vi "AudioTest.SoundCheck Data Log Graph Window - Composite.vi"() -> ()   [LabVIEW 2018]
uses:
  TypeDefs/AudioTest.Analysis Data Record.ctl
  TypeDefs/AudioTest.Analysis Folder Navigation Status.ctl
  <vilib>/KATE/Queues/Queue Utils.lvlib
  <vilib>/KATE/Files/File Utils.lvlib
panel:
  in  "Main Tab":enum32{"Data", "Setup"}(tab)
  out "Comment":string
  out "Count":i32
  out "Index":i32
  out "TopEnd":bool
  out "BotEnd":bool
  out "Loc":string
  out "Result":string
  out "Description":string
  out "Result Code":i32 caption="Code"
  out "Folder":string
  in  "UUTDir Next":bool
  in  "UUTDir Prev":bool
  in  "Snapshot":bool
  out "Name 1 1":string
  out "Graph1 1":cluster{"X":dbl[], "Y":dbl[]}[](graph)
  out "Graph1 2":cluster{"X":dbl[], "Y":dbl[]}[](graph)
  out "Name 1 2":string
  out "Name 3 3":string
  out "Graph3 3":cluster{"X":dbl[], "Y":dbl[]}[](graph)
  out "Name 3 2":string
  out "Graph3 2":cluster{"X":dbl[], "Y":dbl[]}[](graph)
  out "Name 3 1":string
  out "Graph3 1":cluster{"X":dbl[], "Y":dbl[]}[](graph)
  out "Name 2 4":string
  out "Graph2 4":cluster{"X":dbl[], "Y":dbl[]}[](graph)
  out "Graph2 3":cluster{"X":dbl[], "Y":dbl[]}[](graph)
  out "Name 2 3":string
  out "Graph2 2":cluster{"X":dbl[], "Y":dbl[]}[](graph)
  out "Name 2 2":string
  out "Graph2 1":cluster{"X":dbl[], "Y":dbl[]}[](graph)
  out "Name 2 1":string
  out "Graph1 4":cluster{"X":dbl[], "Y":dbl[]}[](graph)
  out "Name 1 4":string
  out "Graph1 3":cluster{"X":dbl[], "Y":dbl[]}[](graph)
  out "Name 1 3":string
  out "Left Level":string caption="Level"
  out "Right Level":string caption="Level"
  out "Mic Level":string caption="Level"
  out "Mic Covered Level":string caption="Covered"
  in  "Graphs":T1[](array[typedef])
  in  "QName":string="Plot_Composite"
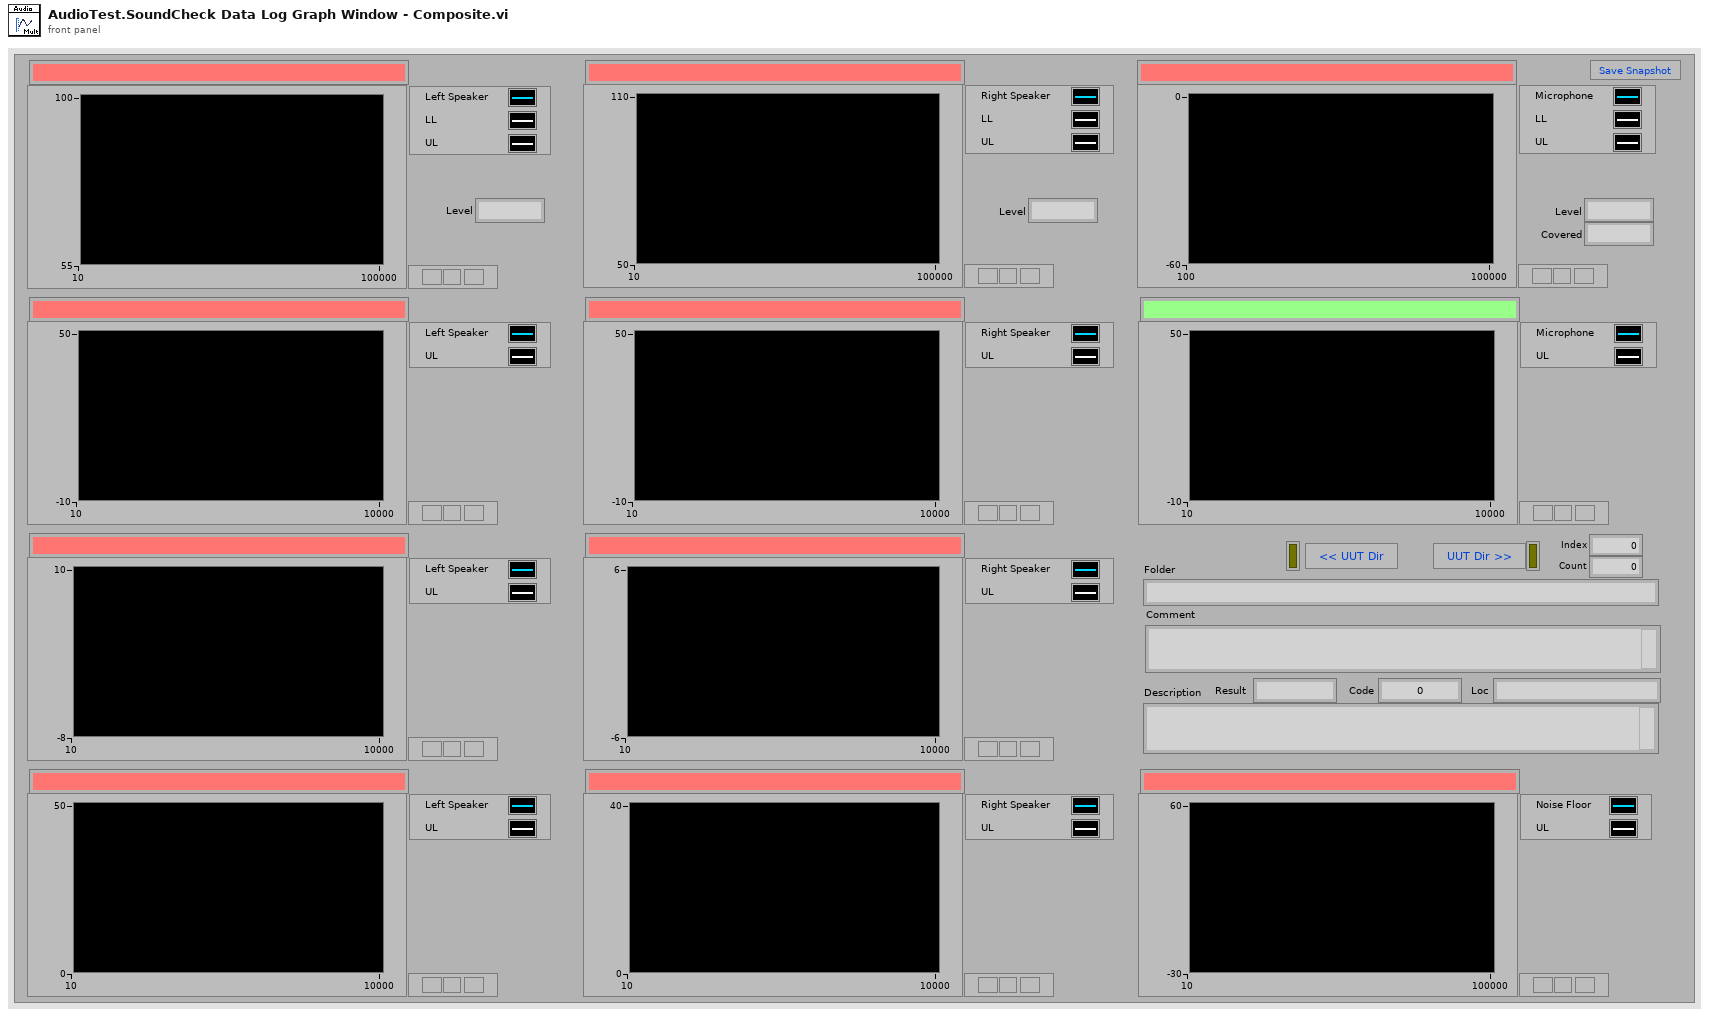
[diagram p1: front panel]
types:
  T1 = typedef "AudioTest.Analysis Data Record.ctl" = cluster{"Name":string, "X Units":string, "Y Units":string, "DataPlots":cluster{"X":dbl[], "Y":dbl[]}[], "LimitPlots":cluster{"X":dbl[], "Y":dbl[]}[], "DataPlotNames":string[], "LimitPlotNames":string[], "Fail":bool}
  T2 = typedef "imagedata.ctl" = cluster{"image type":i32, "image depth":i32, "image":u8[], "mask":u8[], "colors":u32[], "Rectangle":cluster{"left":i16, "top":i16, "right":i16, "bottom":i16}}
  T3 = enum32{"Invalid", "Standard", "Closed", "Hidden", "Minimized", "Maximized"}
  T4 = typedef "AudioTest.Analysis Folder Navigation Status.ctl" = cluster{"Index":i32, "Count":i32, "HightEnd":bool, "LowtEnd":bool}
  T5 = cluster{"Graphs":T1[], "PlotColors":u32[], "LimColors":u32[]}
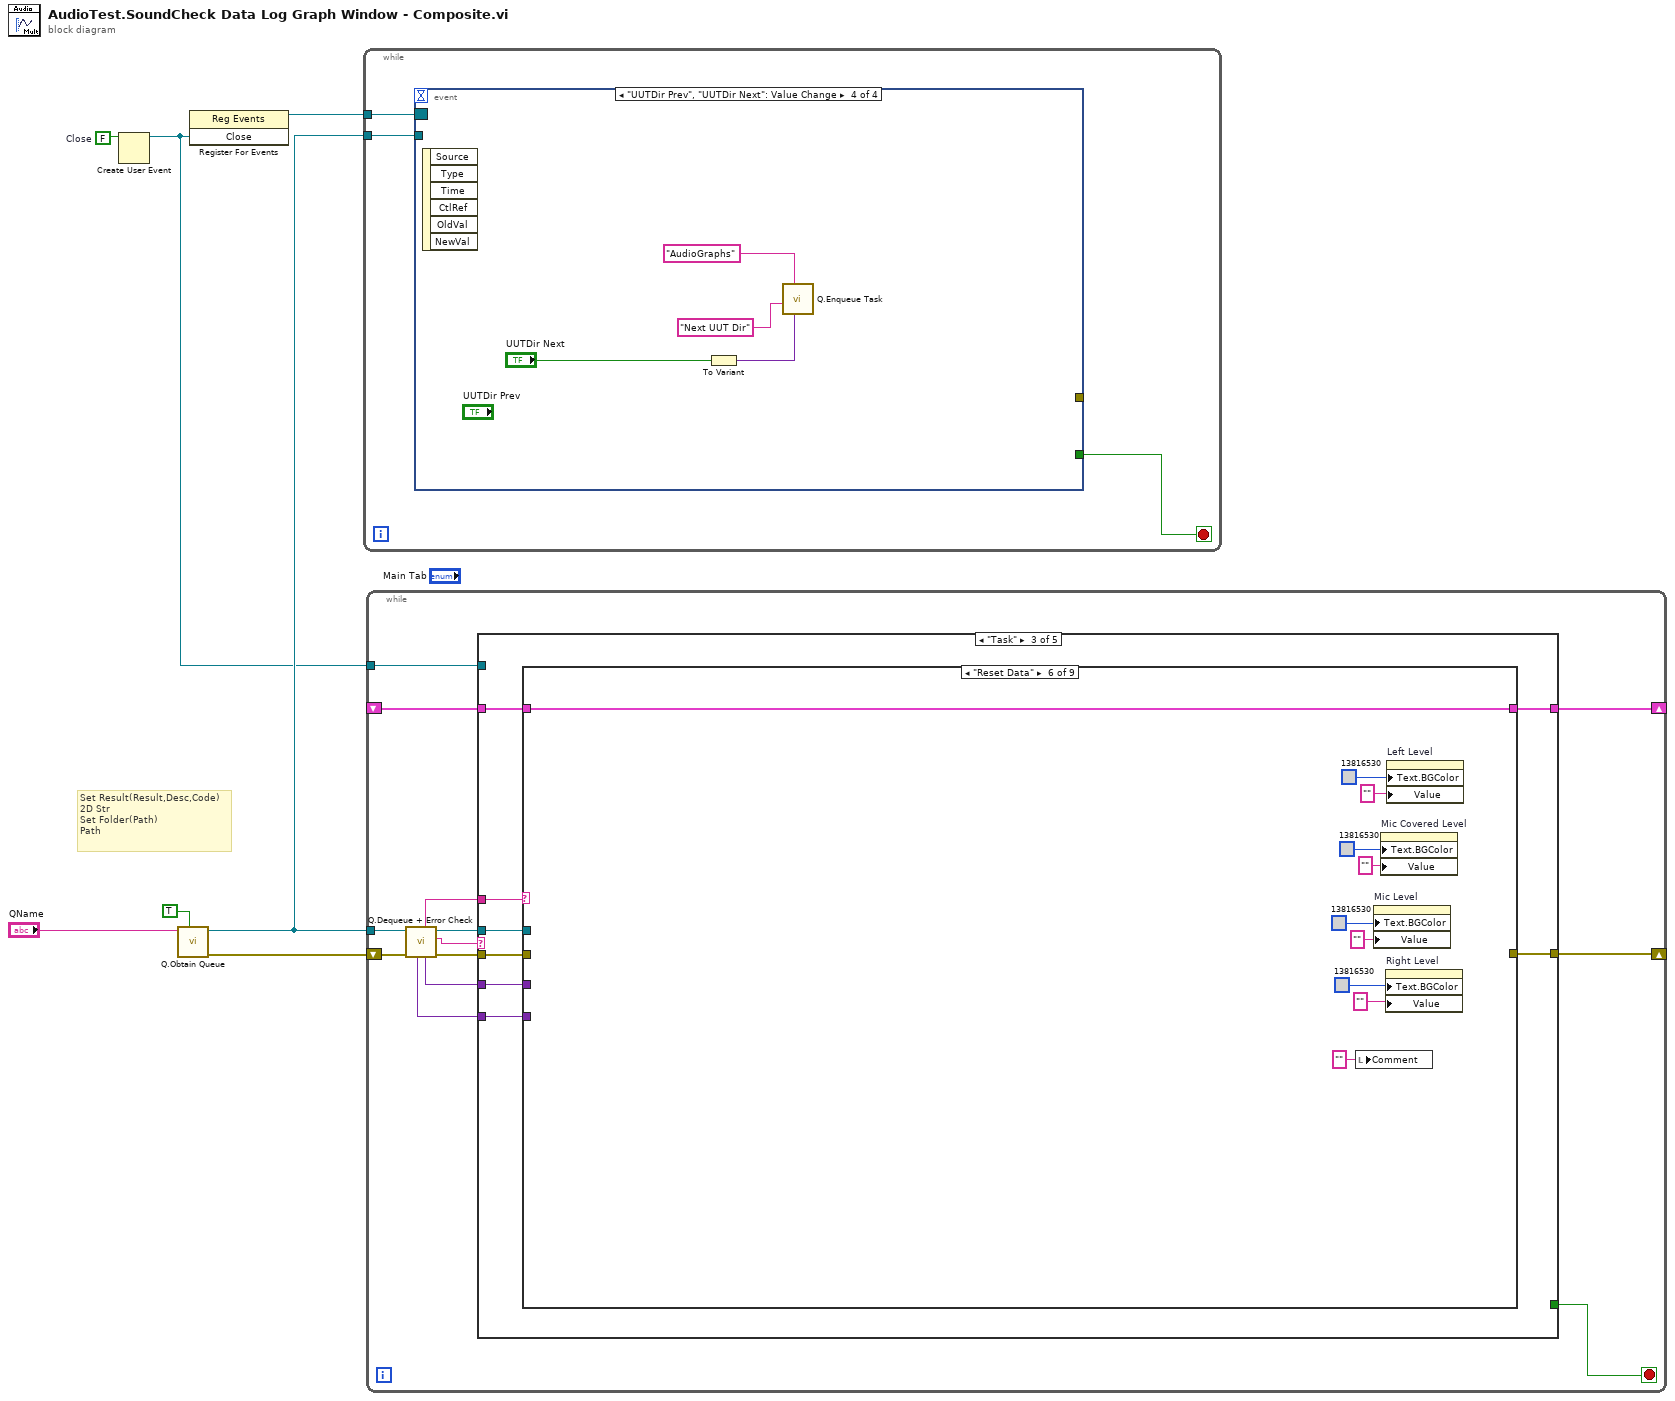
[diagram p0: block diagram]
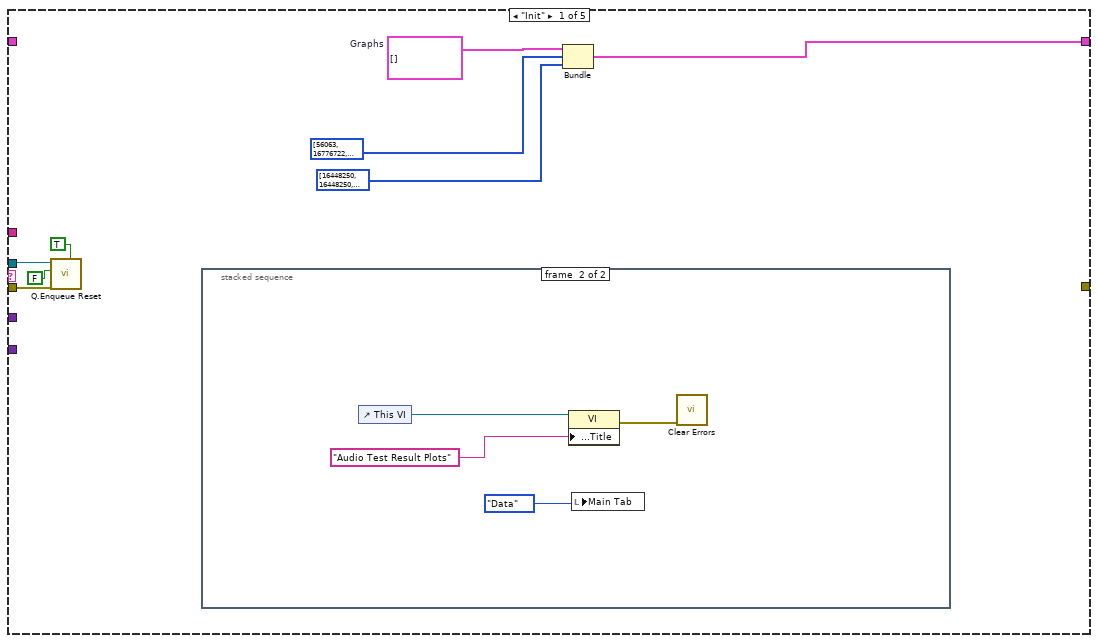
[diagram p2: hidden frame]
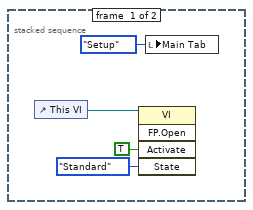
[diagram p3: hidden frame]
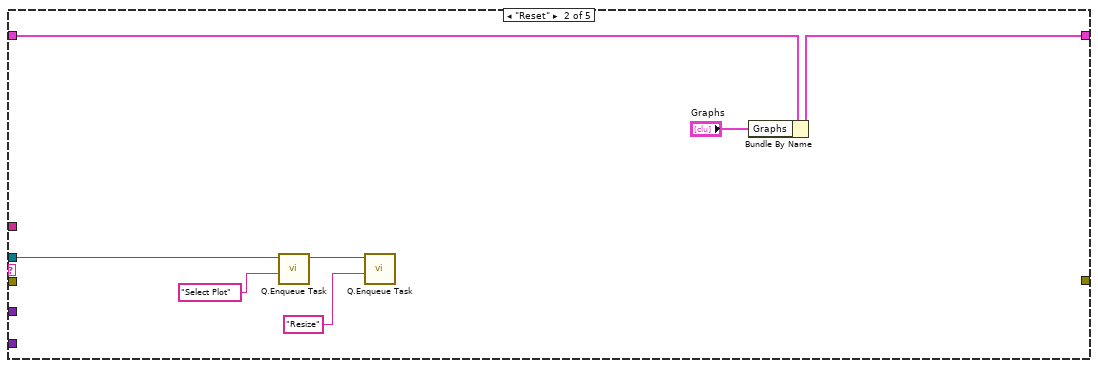
[diagram p4: hidden frame]
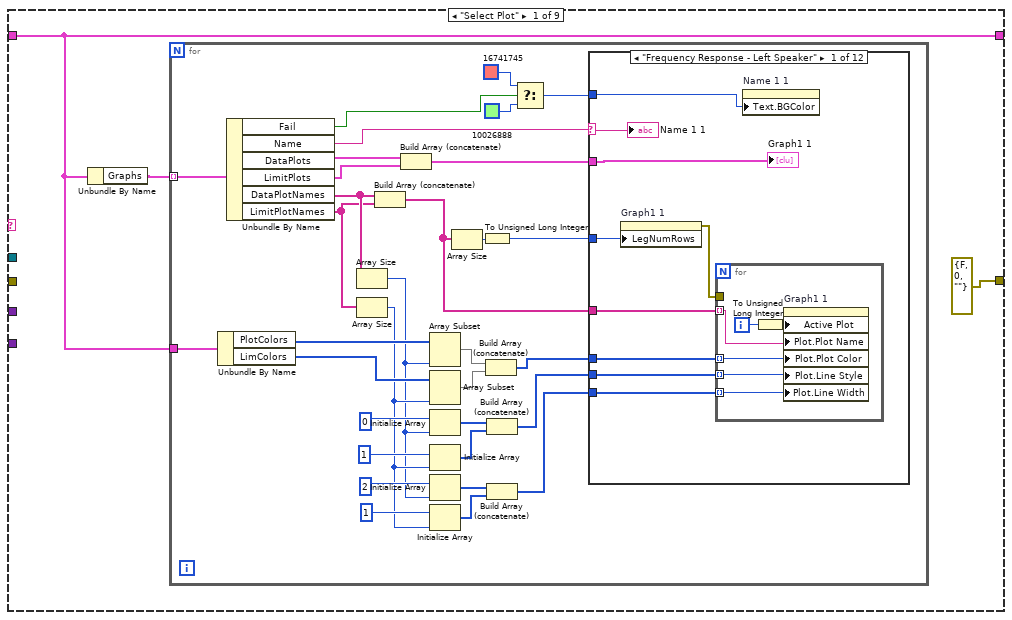
[diagram p5: hidden frame]
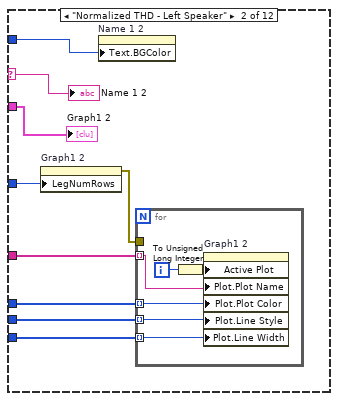
[diagram p6: hidden frame]
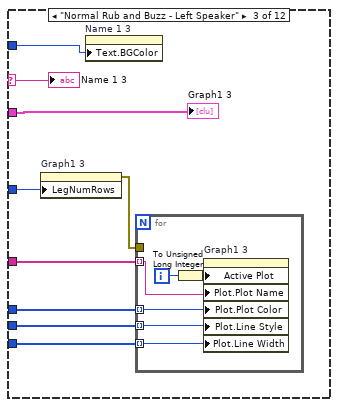
[diagram p7: hidden frame]
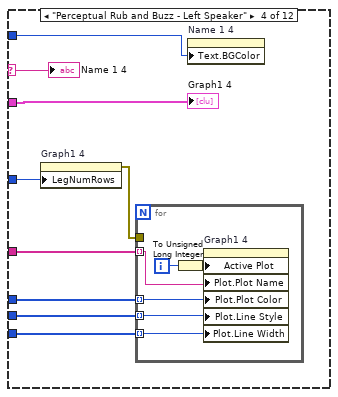
[diagram p8: hidden frame]
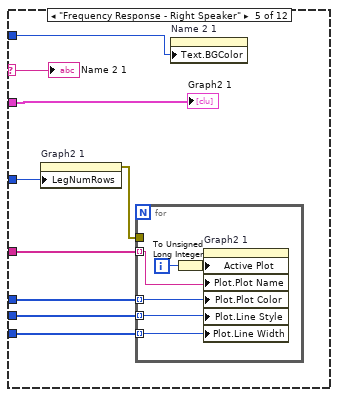
[diagram p9: hidden frame]
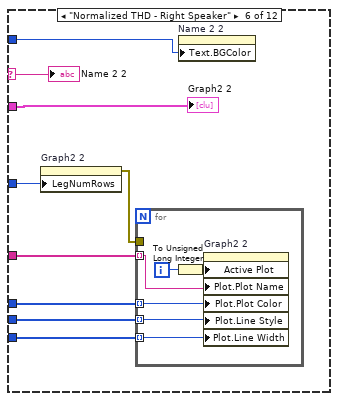
[diagram p10: hidden frame]
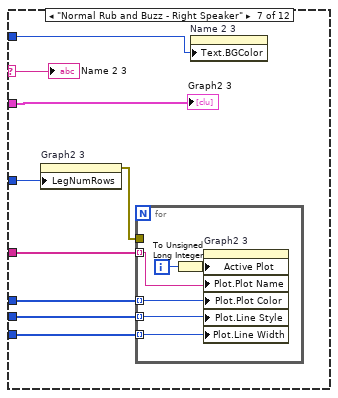
[diagram p11: hidden frame]
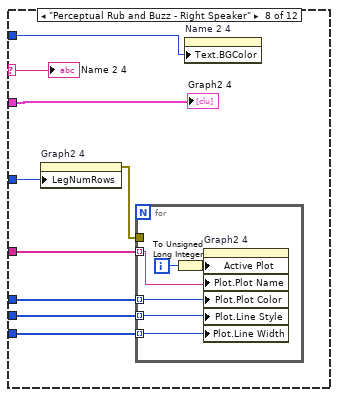
[diagram p12: hidden frame]
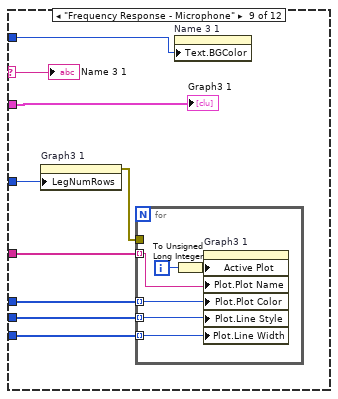
[diagram p13: hidden frame]
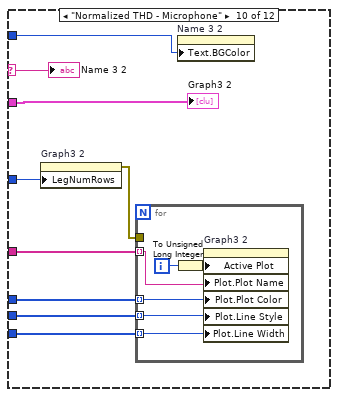
[diagram p14: hidden frame]
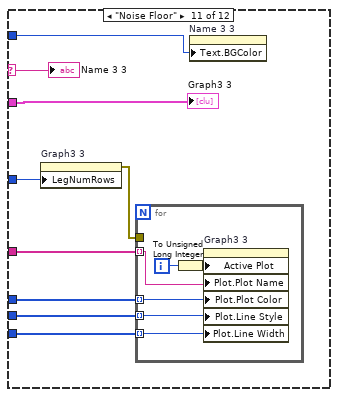
[diagram p15: hidden frame]
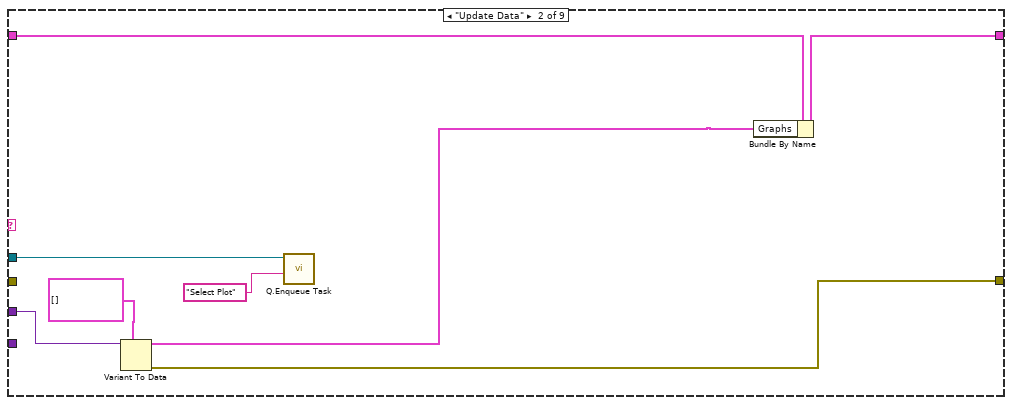
[diagram p17: hidden frame]
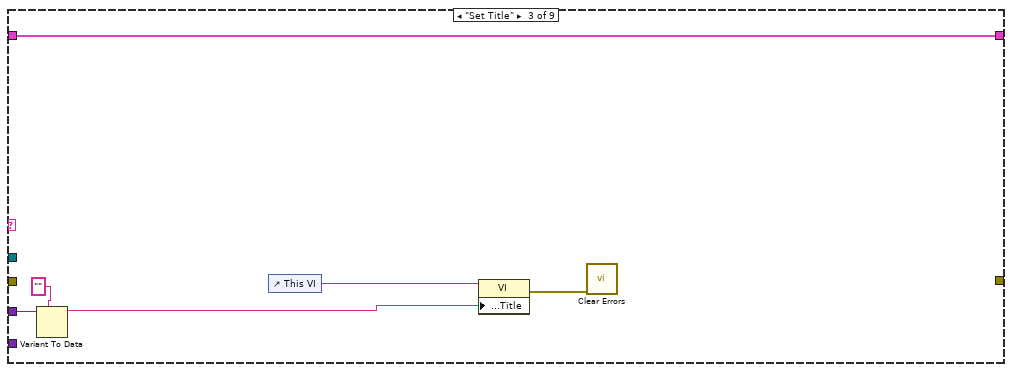
[diagram p18: hidden frame]
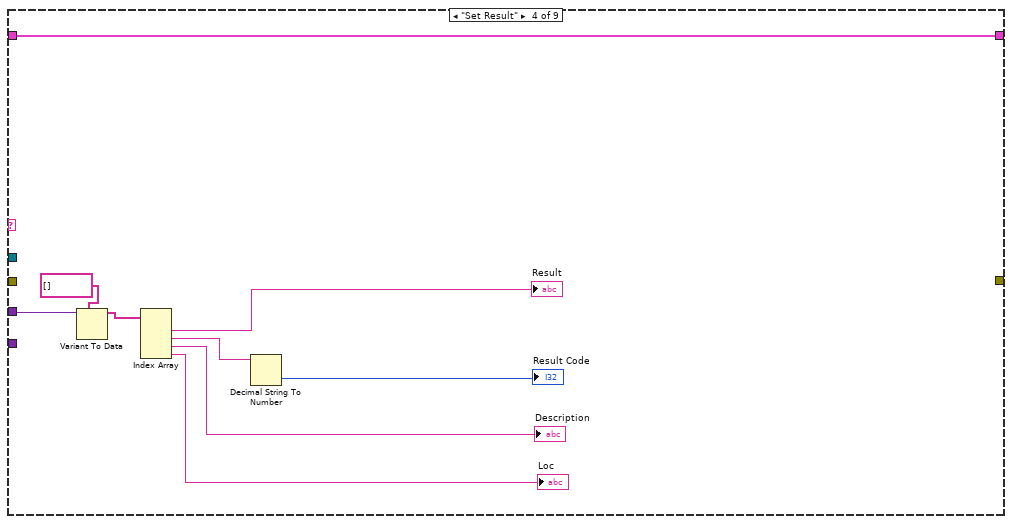
[diagram p19: hidden frame]
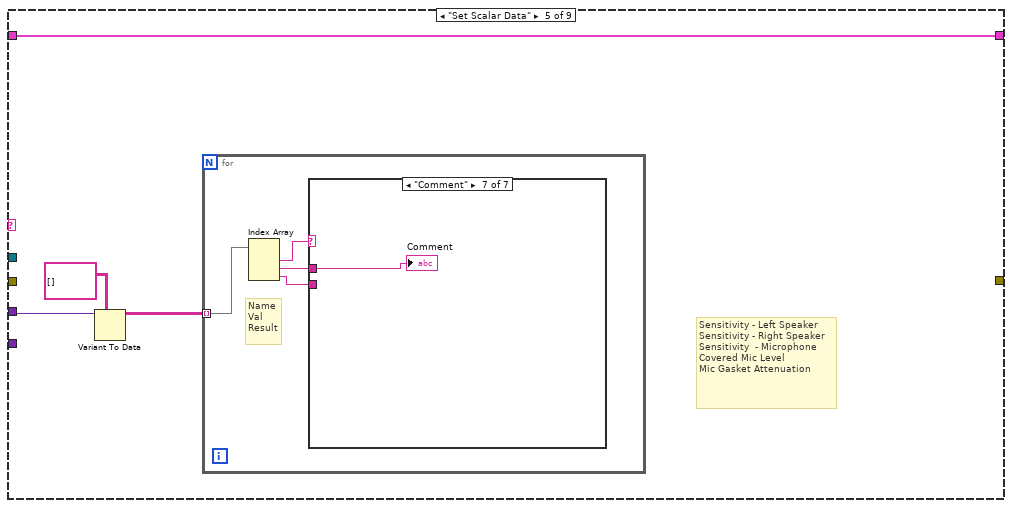
[diagram p20: hidden frame]
diagram:
  w7 = FALSE  # Close
  # "Set Result(Result,Desc,Code)\n2D Str\nSet Folder(Path)\nPath"
  n1 = Create User Event(user event datatype=w7) -> (user event=w2:refnum<user-event>)  [unwired: 1 in, 1 out]
  n2 = call <vilib>:"Q.Obtain Queue.vi"("Enqueue Init"=TRUE, "Q Name"="QName") -> ("error out"=w4:errorcluster, "Q Out"=w3:refnum<queue>)  [unwired: 7 in, 1 out]
  n3 = register-events(w2) -> (reference out=w6:refnum<event-registration>)  [unwired: 2 in, 1 out]
  n4 = while {
    tunnel: w6 -> [w10]
    tunnel: w3 -> [w9]
    stop <- w8 stop-if-true
    n5 = event shown="[3] \"UUTDir Prev\", \"UUTDir Next\": Value Change" {
      selector: w10 -> [_ _ _ _]
      dyn-events: _ -> [_ _ _ _]
      timeout: _ -> [_ _ _ _]
      tunnel: w9 -> [w13 w16 _ _]
      tunnel: [TRUE TRUE _ _] -> w8
      tunnel: [_ _ w23 _] -> _
      event Panel Close? {
        n6 = event-data() -> ()  [unwired: 1 in, 4 out]
        n7 = call <vilib>:"Q.Enqueue Exit.vi"("Q In"=w13) -> ("error out"=w12:errorcluster)  [unwired: 9 in, 1 out]
        n8 = call <vilib>:"Clear Errors.vi"("error in (no error)"=w12) -> ()  [unwired: 5 in, 2 out]
        n9 = event-data("Discard?"=TRUE) -> ()  [unwired: 1 in, 1 out]
      }
      event User Event {
        n10 = event-data() -> ()  [unwired: 1 in, 4 out]
        n11 = call <vilib>:"Q.Enqueue Exit.vi"("Q In"=w16) -> ("error out"=w15:errorcluster)  [unwired: 9 in, 1 out]
        n12 = call <vilib>:"Clear Errors.vi"("error in (no error)"=w15) -> ()  [unwired: 5 in, 2 out]
      }
      event "Snapshot": Value Change {
        n13 = event-data() -> ()  [unwired: 1 in, 6 out]
        n14 = control-ref of="This VI"() -> (w27:refnum<vi>)
        n15 = invoke class="VI" method="FP.Get Image"(reference=w27, "visible area only"=FALSE ("Visible Area Only"), "image depth"=24 ("Image Depth")) -> ("image data"=w24:T2)  [unwired: 3 in, 5 out]
        n16 = call "File Dialog"("prompt"="Select path to save screen shot", "default name"="Audio Graphs.png", "pattern (all files)"="*.png") -> ("selected path"=w22:path, "cancelled"=w18:bool)  [unwired: 9 in, 2 out]
        n17 = case shown="False" w18 {
          tunnel: w24 -> [w30 _]
          tunnel: [w29 _] -> w23
          tunnel: w22 -> [w28 _]
          frame False {
            n18 = call <vilib>:"Write PNG File.vi"("image data"=w30, "path to PNG file"=w28) -> ("error out"=w29:errorcluster)  [unwired: 8 in, 1 out]
          }
          frame True {
          }
        }
      }
      event "UUTDir Prev", "UUTDir Next": Value Change {
        n19 = event-data() -> ()  [unwired: 1 in, 6 out]
        n20 = To Variant(anything="UUTDir Next") -> (Variant=w32:variant)
        n21 = call <vilib>:"Q.Enqueue Task.vi"("Data1"=w32, "Q Name"="AudioGraphs", "Task Name"="Next UUT Dir") -> ()  [unwired: 7 in, 2 out]
      }
    }
  }
  n22 = while {
    shift-right: [w39] -> _
    shift-left: w4 -> [w44]
    tunnel: w3 -> [w42]
    shift-right: [w37] -> _
    shift-left: _ -> [w36]
    tunnel: w2 -> [w35]
    stop <- w38 stop-if-true
    n23 = call <vilib>:"Q.Dequeue + Error Check.vi"("Error In"=w44, "Q In"=w42) -> ("error out"=w45:errorcluster, "Cmd"=w47:string, "Q Out"=w46:refnum<queue>, "Data1"=w41:variant, "Sub"=w43:string, "Data2"=w40:variant)  [unwired: 4 in]
    n24 = case shown="\"Task\"" w47 {
      tunnel: w46 -> [w55 w68 w77 _ w372]
      tunnel: w45 -> [w54 _ w76 _ _]
      tunnel: w43 -> [_ _ w78 _ _]
      tunnel: w41 -> [_ _ w75 _ _]
      tunnel: w40 -> [_ _ w74 _ _]
      tunnel: [_ _ w71 _ _] -> w39
      tunnel: [_ _ _ _ TRUE] -> w38
      tunnel: [w49 w70 w72 w369 w376] -> w37
      tunnel: w36 -> [_ w69 w73 w370 w376]
      tunnel: w35 -> [_ _ _ _ w375]
      frame "Init" {
        w52 = T1[] []  # Graphs
        n25 = call <vilib>:"Q.Enqueue Reset.vi"("Top of Q(T)"=TRUE, "Error In"=w54, "Flush Queue(T)"=FALSE, "Q In"=w55) -> ()  [unwired: 6 in, 2 out]
        n26 = stacked-sequence {
          frame #0 {
            n27 = control-ref of="This VI"() -> (w59:refnum<vi>)
            n28 = invoke class="VI" method="FP.Open"(reference=w59, "Activate"=TRUE ("Activate?"), "State"=T3."Standard") -> ()  [unwired: 2 in, 5 out]
            n29 = local write "Main Tab"(enum32{"Data", "Setup"}."Setup" ("Main Tab")) -> ()
          }
          frame #1 {
            n30 = control-ref of="This VI"() -> (w63:refnum<vi>)
            n31 = property class="VI"(reference=w63, "Front Panel.Title"="Audio Test Result Plots") -> (error out=w62:errorcluster)  [unwired: 1 in, 1 out]
            n32 = local write "Main Tab"(enum32{"Data", "Setup"}."Data" ("Main Tab")) -> ()
            n33 = call <vilib>:"Clear Errors.vi"("error in (no error)"=w62) -> ()  [unwired: 5 in, 2 out]
          }
        }
        n34 = Bundle("Graphs"=w52, "PlotColors"=u32[] [56063, 16776722, 16730898, 16711925, 6618880], "LimColors"=u32[] [16448250, 16448250, 16448250, 16448250, 16448250, 16448250]) -> (w49:T5)  [unwired: 1 in]
      }
      frame "Reset" {
        n35 = call <vilib>:"Q.Enqueue Task.vi"("Task Name"="Select Plot", "Q In"=w68) -> ("Q Out"=w65:refnum<queue>)  [unwired: 8 in, 1 out]
        n36 = call <vilib>:"Q.Enqueue Task.vi"("Task Name"="Resize", "Q In"=w65) -> ()  [unwired: 8 in, 2 out]
        n37 = Bundle By Name(cluster=w69, "Graphs"="Graphs") -> (w70:T5)
      }
      frame "Task" {
        n38 = case shown="\"Reset Data\"" w78 {
          tunnel: w77 -> [_ w285 _ _ _ _ _ _ _]
          tunnel: w76 -> [_ _ _ _ _ _ _ _ _]
          tunnel: w75 -> [_ w282 w289 w300 w302 _ w346 w363 _]
          tunnel: w74 -> [_ _ _ _ _ _ _ _ _]
          tunnel: w73 -> [w81 w284 w292 w301 w305 w340 w347 w365 w366]
          tunnel: [w81 w283 w292 w301 w305 w340 w347 w365 w366] -> w72
          tunnel: [errorcluster {"status"=FALSE, "code"=0, "source"=""} ("error constant") w281 _ _ _ _ _ _ _] -> w71
          frame "Select Plot" {
            n39 = Unbundle By Name(w81) -> ("Graphs"=w79:T1[])
            n40 = for {
              tunnel: w81 -> [w108]
              tunnel: w79 -> [w87] mode=indexing
              n41 = Unbundle By Name(w108) -> ("PlotColors"=w105:u32[], "LimColors"=w104:u32[])
              n42 = Unbundle By Name(w87) -> ("Fail"=w83:bool, "Name"=w86:string, "DataPlots"=w113:cluster{"X":dbl[], "Y":dbl[]}[], "LimitPlots"=w112:cluster{"X":dbl[], "Y":dbl[]}[], "DataPlotNames"=w107:string[], "LimitPlotNames"=w106:string[])
              n43 = Array Size(array=w107) -> (size(s)=w90:i32)
              n44 = Array Size(array=w106) -> (size(s)=w91:i32)
              n45 = Build Array (concatenate)(w107, w106) -> (w109:string[])
              n46 = Build Array (concatenate)(w113, w112) -> (w88:cluster{"X":dbl[], "Y":dbl[]}[])
              n47 = Array Subset(array=w105, length=w90) -> (w103:u32[])  [unwired: 1 in]
              n48 = Array Subset(array=w104, length=w91) -> (w102:u32[])  [unwired: 1 in]
              n49 = Initialize Array(u8 0 ("Plot.Line Style"), w90) -> (w98:u8[])
              n50 = Initialize Array(u8 1 ("Plot.Line Style"), w91) -> (w97:u8[])
              n51 = Initialize Array(u8 2 ("Plot.Line Style"), w90) -> (w94:u8[])
              n52 = Initialize Array(u8 1 ("Plot.Line Style"), w91) -> (w95:u8[])
              n53 = Array Size(array=w109) -> (size(s)=w111:i32)
              n54 = To Unsigned Long Integer(number=w111) -> (unsigned 32bit integer=w110:u32)
              n55 = Build Array (concatenate)(w103, w102) -> (w101:u32[])
              n56 = Build Array (concatenate)(w98, w97) -> (w96:u8[])
              n57 = Build Array (concatenate)(w94, w95) -> (w89:u8[])
              n58 = Select(t=u32 16741745, s=w83, f=u32 10026888) -> (s? t:f=w82:u32)
              n59 = case shown="\"Frequency Response - Left Speaker\"" w86 {
                selector: w86 -> [w115 w130 w145 w160 w175 w190 w205 w220 w235 w250 w265 _]
                tunnel: w110 -> [w122 w137 w152 w167 w182 w197 w212 w227 w242 w257 w272 _]
                tunnel: w109 -> [w120 w135 w150 w165 w180 w195 w210 w225 w240 w255 w270 _]
                tunnel: w101 -> [w119 w134 w149 w164 w179 w194 w209 w224 w239 w254 w269 _]
                tunnel: w96 -> [w118 w133 w148 w163 w178 w193 w208 w223 w238 w253 w268 _]
                tunnel: w89 -> [w117 w132 w147 w162 w177 w192 w207 w222 w237 w252 w267 _]
                tunnel: w88 -> [w116 w131 w146 w161 w176 w191 w206 w221 w236 w251 w266 _]
                tunnel: w82 -> [w114 w129 w144 w159 w174 w189 w204 w219 w234 w249 w264 _]
                frame "Frequency Response - Left Speaker" {
                  n60 = property on="Graph1 1" class="XYGraph (strict)"("LegNumRows"=w122) -> (error out=w121:errorcluster)  [unwired: 2 in, 1 out]
                  n61 = for {
                    tunnel: w120 -> [w126] mode=indexing
                    tunnel: w121 -> [_]
                    tunnel: w119 -> [w125] mode=indexing
                    tunnel: w118 -> [w124] mode=indexing
                    tunnel: w117 -> [w123] mode=indexing
                    i -> [w127]
                    n62 = To Unsigned Long Integer(number=w127) -> (unsigned 32bit integer=w128:u32)
                    n63 = property on="Graph1 1" class="XYGraph (strict)"("Active Plot"=w128, "Plot.Plot Name"=w126, "Plot.Plot Color"=w125, "Plot.Line Style"=w124, "Plot.Line Width"=w123) -> ()  [unwired: 2 in, 2 out]
                  }
                  n64 = property on="Name 1 1" class="Str"("Text.BGColor"=w114) -> ()  [unwired: 2 in, 2 out]
                  "Graph1 1" <- w116
                  "Name 1 1" <- w115
                }
                frame "Normalized THD - Left Speaker" {
                  n65 = property on="Graph1 2" class="XYGraph (strict)"("LegNumRows"=w137) -> (error out=w136:errorcluster)  [unwired: 2 in, 1 out]
                  n66 = property on="Name 1 2" class="Str"("Text.BGColor"=w129) -> ()  [unwired: 2 in, 2 out]
                  n67 = for {
                    tunnel: w135 -> [w141] mode=indexing
                    tunnel: w136 -> [_]
                    tunnel: w134 -> [w140] mode=indexing
                    tunnel: w133 -> [w139] mode=indexing
                    tunnel: w132 -> [w138] mode=indexing
                    i -> [w142]
                    n68 = To Unsigned Long Integer(number=w142) -> (unsigned 32bit integer=w143:u32)
                    n69 = property on="Graph1 2" class="XYGraph (strict)"("Active Plot"=w143, "Plot.Plot Name"=w141, "Plot.Plot Color"=w140, "Plot.Line Style"=w139, "Plot.Line Width"=w138) -> ()  [unwired: 2 in, 2 out]
                  }
                  "Graph1 2" <- w131
                  "Name 1 2" <- w130
                }
                frame "Normal Rub and Buzz - Left Speaker" {
                  n70 = property on="Graph1 3" class="XYGraph (strict)"("LegNumRows"=w152) -> (error out=w151:errorcluster)  [unwired: 2 in, 1 out]
                  n71 = property on="Name 1 3" class="Str"("Text.BGColor"=w144) -> ()  [unwired: 2 in, 2 out]
                  n72 = for {
                    tunnel: w150 -> [w156] mode=indexing
                    tunnel: w151 -> [_]
                    tunnel: w149 -> [w155] mode=indexing
                    tunnel: w148 -> [w154] mode=indexing
                    tunnel: w147 -> [w153] mode=indexing
                    i -> [w157]
                    n73 = To Unsigned Long Integer(number=w157) -> (unsigned 32bit integer=w158:u32)
                    n74 = property on="Graph1 3" class="XYGraph (strict)"("Active Plot"=w158, "Plot.Plot Name"=w156, "Plot.Plot Color"=w155, "Plot.Line Style"=w154, "Plot.Line Width"=w153) -> ()  [unwired: 2 in, 2 out]
                  }
                  "Graph1 3" <- w146
                  "Name 1 3" <- w145
                }
                frame "Perceptual Rub and Buzz - Left Speaker" {
                  n75 = property on="Graph1 4" class="XYGraph (strict)"("LegNumRows"=w167) -> (error out=w166:errorcluster)  [unwired: 2 in, 1 out]
                  n76 = for {
                    tunnel: w165 -> [w171] mode=indexing
                    tunnel: w166 -> [_]
                    tunnel: w164 -> [w170] mode=indexing
                    tunnel: w163 -> [w169] mode=indexing
                    tunnel: w162 -> [w168] mode=indexing
                    i -> [w172]
                    n77 = To Unsigned Long Integer(number=w172) -> (unsigned 32bit integer=w173:u32)
                    n78 = property on="Graph1 4" class="XYGraph (strict)"("Active Plot"=w173, "Plot.Plot Name"=w171, "Plot.Plot Color"=w170, "Plot.Line Style"=w169, "Plot.Line Width"=w168) -> ()  [unwired: 2 in, 2 out]
                  }
                  n79 = property on="Name 1 4" class="Str"("Text.BGColor"=w159) -> ()  [unwired: 2 in, 2 out]
                  "Graph1 4" <- w161
                  "Name 1 4" <- w160
                }
                frame "Frequency Response - Right Speaker" {
                  n80 = property on="Graph2 1" class="XYGraph (strict)"("LegNumRows"=w182) -> (error out=w181:errorcluster)  [unwired: 2 in, 1 out]
                  n81 = for {
                    tunnel: w180 -> [w186] mode=indexing
                    tunnel: w181 -> [_]
                    tunnel: w179 -> [w185] mode=indexing
                    tunnel: w178 -> [w184] mode=indexing
                    tunnel: w177 -> [w183] mode=indexing
                    i -> [w187]
                    n82 = To Unsigned Long Integer(number=w187) -> (unsigned 32bit integer=w188:u32)
                    n83 = property on="Graph2 1" class="XYGraph (strict)"("Active Plot"=w188, "Plot.Plot Name"=w186, "Plot.Plot Color"=w185, "Plot.Line Style"=w184, "Plot.Line Width"=w183) -> ()  [unwired: 2 in, 2 out]
                  }
                  n84 = property on="Name 2 1" class="Str"("Text.BGColor"=w174) -> ()  [unwired: 2 in, 2 out]
                  "Graph2 1" <- w176
                  "Name 2 1" <- w175
                }
                frame "Normalized THD - Right Speaker" {
                  n85 = property on="Graph2 2" class="XYGraph (strict)"("LegNumRows"=w197) -> (error out=w196:errorcluster)  [unwired: 2 in, 1 out]
                  n86 = for {
                    tunnel: w195 -> [w201] mode=indexing
                    tunnel: w196 -> [_]
                    tunnel: w194 -> [w200] mode=indexing
                    tunnel: w193 -> [w199] mode=indexing
                    tunnel: w192 -> [w198] mode=indexing
                    i -> [w202]
                    n87 = To Unsigned Long Integer(number=w202) -> (unsigned 32bit integer=w203:u32)
                    n88 = property on="Graph2 2" class="XYGraph (strict)"("Active Plot"=w203, "Plot.Plot Name"=w201, "Plot.Plot Color"=w200, "Plot.Line Style"=w199, "Plot.Line Width"=w198) -> ()  [unwired: 2 in, 2 out]
                  }
                  n89 = property on="Name 2 2" class="Str"("Text.BGColor"=w189) -> ()  [unwired: 2 in, 2 out]
                  "Graph2 2" <- w191
                  "Name 2 2" <- w190
                }
                frame "Normal Rub and Buzz - Right Speaker" {
                  n90 = property on="Graph2 3" class="XYGraph (strict)"("LegNumRows"=w212) -> (error out=w211:errorcluster)  [unwired: 2 in, 1 out]
                  n91 = for {
                    tunnel: w210 -> [w216] mode=indexing
                    tunnel: w211 -> [_]
                    tunnel: w209 -> [w215] mode=indexing
                    tunnel: w208 -> [w214] mode=indexing
                    tunnel: w207 -> [w213] mode=indexing
                    i -> [w217]
                    n92 = To Unsigned Long Integer(number=w217) -> (unsigned 32bit integer=w218:u32)
                    n93 = property on="Graph2 3" class="XYGraph (strict)"("Active Plot"=w218, "Plot.Plot Name"=w216, "Plot.Plot Color"=w215, "Plot.Line Style"=w214, "Plot.Line Width"=w213) -> ()  [unwired: 2 in, 2 out]
                  }
                  n94 = property on="Name 2 3" class="Str"("Text.BGColor"=w204) -> ()  [unwired: 2 in, 2 out]
                  "Graph2 3" <- w206
                  "Name 2 3" <- w205
                }
                frame "Perceptual Rub and Buzz - Right Speaker" {
                  n95 = property on="Graph2 4" class="XYGraph (strict)"("LegNumRows"=w227) -> (error out=w226:errorcluster)  [unwired: 2 in, 1 out]
                  n96 = for {
                    tunnel: w225 -> [w231] mode=indexing
                    tunnel: w226 -> [_]
                    tunnel: w224 -> [w230] mode=indexing
                    tunnel: w223 -> [w229] mode=indexing
                    tunnel: w222 -> [w228] mode=indexing
                    i -> [w232]
                    n97 = To Unsigned Long Integer(number=w232) -> (unsigned 32bit integer=w233:u32)
                    n98 = property on="Graph2 4" class="XYGraph (strict)"("Active Plot"=w233, "Plot.Plot Name"=w231, "Plot.Plot Color"=w230, "Plot.Line Style"=w229, "Plot.Line Width"=w228) -> ()  [unwired: 2 in, 2 out]
                  }
                  n99 = property on="Name 2 4" class="Str"("Text.BGColor"=w219) -> ()  [unwired: 2 in, 2 out]
                  "Graph2 4" <- w221
                  "Name 2 4" <- w220
                }
                frame "Frequency Response - Microphone" {
                  n100 = property on="Graph3 1" class="XYGraph (strict)"("LegNumRows"=w242) -> (error out=w241:errorcluster)  [unwired: 2 in, 1 out]
                  n101 = for {
                    tunnel: w240 -> [w246] mode=indexing
                    tunnel: w241 -> [_]
                    tunnel: w239 -> [w245] mode=indexing
                    tunnel: w238 -> [w244] mode=indexing
                    tunnel: w237 -> [w243] mode=indexing
                    i -> [w247]
                    n102 = To Unsigned Long Integer(number=w247) -> (unsigned 32bit integer=w248:u32)
                    n103 = property on="Graph3 1" class="XYGraph (strict)"("Active Plot"=w248, "Plot.Plot Name"=w246, "Plot.Plot Color"=w245, "Plot.Line Style"=w244, "Plot.Line Width"=w243) -> ()  [unwired: 2 in, 2 out]
                  }
                  n104 = property on="Name 3 1" class="Str"("Text.BGColor"=w234) -> ()  [unwired: 2 in, 2 out]
                  "Graph3 1" <- w236
                  "Name 3 1" <- w235
                }
                frame "Normalized THD - Microphone" {
                  n105 = property on="Graph3 2" class="XYGraph (strict)"("LegNumRows"=w257) -> (error out=w256:errorcluster)  [unwired: 2 in, 1 out]
                  n106 = for {
                    tunnel: w255 -> [w261] mode=indexing
                    tunnel: w256 -> [_]
                    tunnel: w254 -> [w260] mode=indexing
                    tunnel: w253 -> [w259] mode=indexing
                    tunnel: w252 -> [w258] mode=indexing
                    i -> [w262]
                    n107 = To Unsigned Long Integer(number=w262) -> (unsigned 32bit integer=w263:u32)
                    n108 = property on="Graph3 2" class="XYGraph (strict)"("Active Plot"=w263, "Plot.Plot Name"=w261, "Plot.Plot Color"=w260, "Plot.Line Style"=w259, "Plot.Line Width"=w258) -> ()  [unwired: 2 in, 2 out]
                  }
                  n109 = property on="Name 3 2" class="Str"("Text.BGColor"=w249) -> ()  [unwired: 2 in, 2 out]
                  "Graph3 2" <- w251
                  "Name 3 2" <- w250
                }
                frame "Noise Floor" {
                  n110 = property on="Graph3 3" class="XYGraph (strict)"("LegNumRows"=w272) -> (error out=w271:errorcluster)  [unwired: 2 in, 1 out]
                  n111 = for {
                    tunnel: w270 -> [w276] mode=indexing
                    tunnel: w271 -> [_]
                    tunnel: w269 -> [w275] mode=indexing
                    tunnel: w268 -> [w274] mode=indexing
                    tunnel: w267 -> [w273] mode=indexing
                    i -> [w277]
                    n112 = To Unsigned Long Integer(number=w277) -> (unsigned 32bit integer=w278:u32)
                    n113 = property on="Graph3 3" class="XYGraph (strict)"("Active Plot"=w278, "Plot.Plot Name"=w276, "Plot.Plot Color"=w275, "Plot.Line Style"=w274, "Plot.Line Width"=w273) -> ()  [unwired: 2 in, 2 out]
                  }
                  n114 = property on="Name 3 3" class="Str"("Text.BGColor"=w264) -> ()  [unwired: 2 in, 2 out]
                  "Graph3 3" <- w266
                  "Name 3 3" <- w265
                }
                frame Default {
                }
              }
            }
          }
          frame "Update Data" {
            n115 = Variant To Data(type=T1[] [] ("Graphs"), Variant=w282) -> (data=w280:T1[], error out=w281:errorcluster)  [unwired: 1 in]
            n116 = call <vilib>:"Q.Enqueue Task.vi"("Task Name"="Select Plot", "Q In"=w285) -> ()  [unwired: 8 in, 2 out]
            n117 = Bundle By Name(cluster=w284, "Graphs"=w280) -> (w283:T5)
          }
          frame "Set Title" {
            n118 = Variant To Data(type="", Variant=w289) -> (data=w287:string)  [unwired: 1 in, 1 out]
            n119 = control-ref of="This VI"() -> (w291:refnum<vi>)
            n120 = property class="VI"(reference=w291, "Front Panel.Title"=w287) -> (error out=w290:errorcluster)  [unwired: 1 in, 1 out]
            n121 = call <vilib>:"Clear Errors.vi"("error in (no error)"=w290) -> ()  [unwired: 5 in, 2 out]
          }
          frame "Set Result" {
            n122 = Variant To Data(type=string[] [], Variant=w300) -> (data=w298:string[])  [unwired: 1 in, 1 out]
            n123 = Index Array(array=w298) -> (element #1=→"Result":string, element #2=w295:string, element #3=→"Description":string, element #4=→"Loc":string)  [unwired: 4 in]
            n124 = Decimal String To Number(string=w295) -> (number=→"Result Code":i32)  [unwired: 2 in, 1 out]
          }
          frame "Set Scalar Data" {
            # "Sensitivity - Left Speaker\nSensitivity - Right Speaker\nSensitivity  - Microphone\nCovered Mic Level\nMic Gasket Attenuation"
            n125 = Variant To Data(type=string[][] [], Variant=w302) -> (data=w303:string[][])  [unwired: 1 in, 1 out]
            n126 = for {
              tunnel: w303 -> [w309] mode=indexing
              # "Name\nVal\nResult"
              n127 = Index Array(array=w309) -> (element #1=w308:string, element #2=w307:string, element #3=w306:string)  [unwired: 3 in]
              n128 = case shown="\"Comment\"" w308 {
                tunnel: w307 -> [_ w310 w315 w320 w325 _ w330]
                tunnel: w306 -> [_ w312 w317 w322 _ w327 _]
                frame Default {
                }
                frame "Sensitivity - Left Speaker" {
                  n129 = case shown="\"FAIL\"" w312 {
                    tunnel: [u32 13816530 u32 16753568] -> w311
                    frame Default {
                    }
                    frame "FAIL" {
                    }
                  }
                  n130 = property on="Left Level" class="Str"("Text.BGColor"=w311) -> ()  [unwired: 2 in, 2 out]
                  "Left Level" <- w310
                }
                frame "Sensitivity - Right Speaker" {
                  n131 = case shown="\"FAIL\"" w317 {
                    tunnel: [u32 13816530 u32 16753568] -> w316
                    frame Default {
                    }
                    frame "FAIL" {
                    }
                  }
                  n132 = property on="Right Level" class="Str"("Text.BGColor"=w316) -> ()  [unwired: 2 in, 2 out]
                  "Right Level" <- w315
                }
                frame "Sensitivity  - Microphone" {
                  n133 = case shown="Default" w322 {
                    tunnel: [u32 13816530 u32 16753568] -> w321
                    frame Default {
                    }
                    frame "FAIL" {
                    }
                  }
                  n134 = property on="Mic Level" class="Str"("Text.BGColor"=w321) -> ()  [unwired: 2 in, 2 out]
                  "Mic Level" <- w320
                }
                frame "Covered Mic Level" {
                  "Mic Covered Level" <- w325
                }
                frame "Mic Gasket Attenuation" {
                  n135 = case shown="\"FAIL\"" w327 {
                    tunnel: [u32 13816530 u32 16753568] -> w326
                    frame Default {
                    }
                    frame "FAIL" {
                    }
                  }
                  n136 = property on="Mic Covered Level" class="Str"("Text.BGColor"=w326) -> ()  [unwired: 2 in, 2 out]
                }
                frame "Comment" {
                  "Comment" <- w330
                }
              }
            }
          }
          frame "Reset Data" {
            n137 = local write "Comment"("" ("Comment")) -> ()
            n138 = property on="Mic Level" class="Str"("Text.BGColor"=u32 13816530, "Value"="" ("Mic Level")) -> ()  [unwired: 2 in, 2 out]
            n139 = property on="Mic Covered Level" class="Str"("Text.BGColor"=u32 13816530, "Value"="" ("Mic Level")) -> ()  [unwired: 2 in, 2 out]
            n140 = property on="Right Level" class="Str"("Text.BGColor"=u32 13816530, "Value"="" ("Mic Level")) -> ()  [unwired: 2 in, 2 out]
            n141 = property on="Left Level" class="Str"("Text.BGColor"=u32 13816530, "Value"="" ("Mic Level")) -> ()  [unwired: 2 in, 2 out]
          }
          frame "Set Folder" {
            n142 = Variant To Data(type=path "", Variant=w346) -> (data=w343:path)  [unwired: 1 in, 1 out]
            n143 = call <vilib>:"File.Check if File or Folder Exists.vi"("Path"=w343) -> ("Exists"=w341:bool, "Dup Path"=w342:path)  [unwired: 6 in, 3 out]
            n144 = case shown="False" w341 {
              tunnel: w342 -> [_ w354]
              tunnel: ["N/A" ("name") w350] -> w344
              frame False {
              }
              frame True {
                n145 = File/Directory Info(path=w354) -> (path out=w352:path, directory=w353:bool, error out=w349:errorcluster)  [unwired: 1 in, 4 out]
                n146 = case shown="False" w353 {
                  tunnel: w352 -> [w355 w357]
                  tunnel: [w356 w357] -> w351
                  tunnel: w349 -> [_ _]
                  frame False {
                    n147 = Strip Path(path=w355) -> (stripped path=w356:path)  [unwired: 1 out]
                  }
                  frame True {
                  }
                }
                n148 = Strip Path(path=w351) -> (name=w350:string)  [unwired: 1 out]
              }
            }
            "Folder" <- w344
          }
          frame "DirNav" {
            n149 = Variant To Data(type=T4 {"Index"=0, "Count"=0, "HightEnd"=FALSE, "LowtEnd"=FALSE} ("FolderNavStatus"), Variant=w363) -> (data=w362:T4)  [unwired: 1 in, 1 out]
            n150 = Unbundle By Name(w362) -> ("Index"=→"Index":i32, "Count"=→"Count":i32, "HightEnd"=→"TopEnd":bool, "LowtEnd"=→"BotEnd":bool)
          }
          frame Default {
          }
        }
      }
      frame "Error", Default {
        # "Do Nothing (for now)"
        n151 = local write "Graph1 1"(cluster{"X":dbl[], "Y":dbl[]}[] [] ("XY Graph")) -> ()
        n152 = Bundle By Name(cluster=w370, "Graphs"=T1[] []) -> (w369:T5)
      }
      frame "Exit" {
        n153 = Release Queue(queue=w372, force destroy? (F)=TRUE) -> ()  [unwired: 1 in, 3 out]
        n154 = Generate User Event(user event=w375, event data cluster=TRUE ("event data")) -> ()  [unwired: 2 in, 2 out]
        n155 = case shown="True" TRUE {
          tunnel: [_ w378] -> _
          frame False {
          }
          frame True {
            n156 = control-ref of="This VI"() -> (w380:refnum<vi>)
            n157 = invoke class="VI" method="FP.Close"(reference=w380) -> (error out=w379:errorcluster)  [unwired: 2 in, 2 out]
            n158 = Close Reference(reference=w380, error in (no error)=w379) -> (error out=w378:errorcluster)
          }
        }
      }
    }
  }
